vi "DefaultFromIni.vi"(8 "error in (no error)":errorcluster, 11 "RoomAlert in":refnum<class "RoomAlert.lvclass">) -> (0 "error out":errorcluster, 3 "RoomAlert out":refnum<class "RoomAlert.lvclass">)   [LabVIEW 2018, in "SensorPlugins.lvlib" / "RoomAlert.lvclass"]
doc: "Opens the configuration INI file and loads the information from the file into the class cluster."
uses:
  RoomAlert.lvclass
  C:/Program Files (x86)/National Instruments/LabVIEW 2018/user.lib/NIST/BaseClasses/BasePlugin_class/BasePlugin.lvclass
  TypeDefinitions/RoomAlertControls.ctl
  TypeDefinitions/MeasurementControls.ctl
  <userlib>/NIST/BaseClasses/BasePlugin_class/BasePlugin.lvclass/BasePlugin.ctl
  <userlib>/NIST/BaseClasses/BasePlugin_class/Accessors/Read PluginIniFilePath.vi
  <vilib>/Utility/error.llb/Error Cluster From Error Code.vi
  <vilib>/ErrorRing/Error Ring.xnode
  <vilib>/Utility/config.llb/NI_LVConfig.lvlib
  TestClass/Test.lvclass
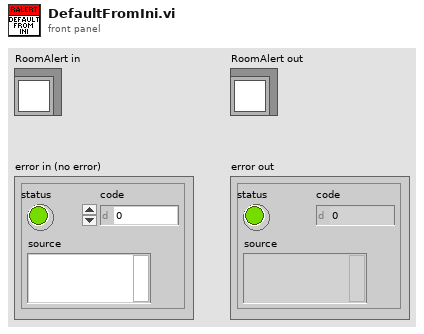
[diagram p1: front panel]
types:
  T1 = typedef "SensorPlugins.lvlib/RoomAlert.lvclass/MeasurementControls.ctl" = cluster{"Measurement RefreshTime (ms)":u32, "Measurement Name":string, "Timeout(ms)":i32, "Amber Warning Light Configuration":cluster{"Warning Temperture (Degrees C)":dbl, "Temperature Delta (Degrees C/Minute)":dbl, "Time Window (Minutes)":dbl}}
  T2 = typedef "SensorPlugins.lvlib/RoomAlert.lvclass/RoomAlertControls.ctl" = cluster{"Connected?":bool, "IP Address of SNMP Device":string, "Port (161)":u16, "Community Name":string, "Measurements To Read Array":u16[], "Update LightTower?":bool, "LightTower":cluster{"Red":bool, "Amber":bool, "Green":bool, "Audio":bool}, "RoomAlert Model ID":string, "Sensor OID Numbers":string[][], "Sensor Light Tower OID Numbers":string[][]}[]
  T3 = typedef "Test.lvclass/INIInfo.ctl" = cluster{"Module Name":string, "INI File Name":string, "Class Name":string, "INI File Name Without Extension":string, "Module.Class.INI File Name":string, "Visualization VI Path":path, "Instrument Class Path":path}
  T4 = typedef "NI_LVConfig.lvlib/Config Data RefNum.ctl" = refnum<k1>
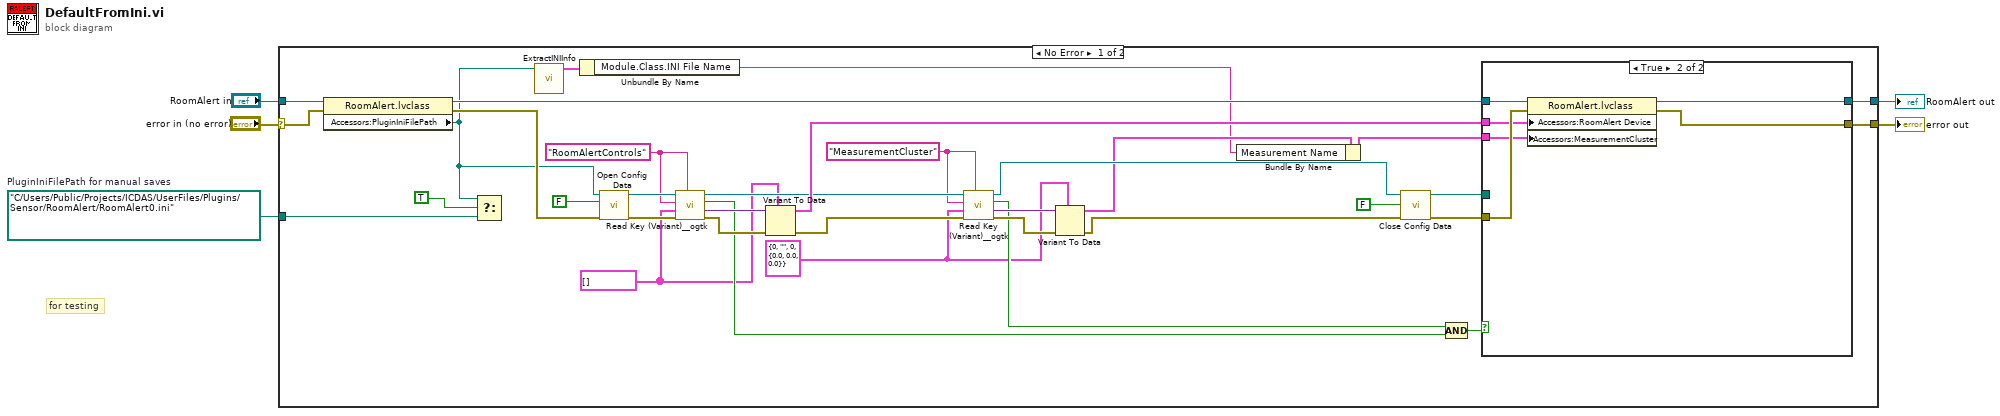
[diagram p0: block diagram]
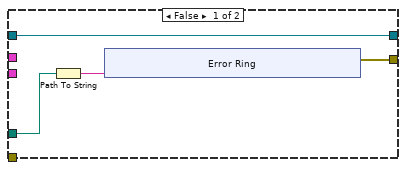
[diagram p2: hidden frame]
diagram:
  w1 = path "C:/Users/Public/Projects/ICDAS/UserFiles/Plugins/Sensor/RoomAlert/RoomAlert0.ini"  # PluginIniFilePath for manual saves
  # "for testing"
  n1 = case shown="No Error" "error in (no error)" {
    selector: "error in (no error)" -> [w39 w58]
    tunnel: "RoomAlert in" -> [w40 w59]
    tunnel: [w34 w59] -> w3
    tunnel: [w30 w58] -> w2
    tunnel: w1 -> [w10 _]
    frame No Error {
      w14 = T1 {"Measurement RefreshTime (ms)"=0, "Measurement Name"="", "Timeout(ms)"=0, "Amber Warning Light Configuration"={"Warning Temperture (Degrees C)"=0.0, "Temperature Delta (Degrees C/Minute)"=0.0, "Time Window (Minutes)"=0.0}} ("MeasurementCluster")
      w15 = T2 [] ("RoomAlert Device")
      w18 = "MeasurementCluster" ("section")
      w27 = "RoomAlertControls" ("section")
      n2 = property class="RoomAlert.lvclass"(reference=w40, error in=w39) -> (reference out=w11:refnum<class "RoomAlert.lvclass">, error out=w37:errorcluster, "Accessors:PluginIniFilePath"=w9:path)
      n3 = Select(t=w9, s=TRUE ("Read from Property Node"), f=w10) -> ()  [unwired: 1 out]
      n4 = call "ExtractINIInfo.vi"("INI File Path"=w9) -> ("INI Info"=w7:T3)  [unwired: 4 in, 6 out]
      n5 = Unbundle By Name(w7) -> ("Module.Class.INI File Name"=w6:string)
      n6 = call <vilib>:"Open Config Data.vi"("error in (no error)"=w37, "create file if necessary (T)"=FALSE, "configuration file path"=w9) -> ("error out"=w35:errorcluster, "refnum"=w36:T4)  [unwired: 6 in, 1 out]
      n7 = call <userlib>:"Read Key (Variant)__ogtk.vi"("section"=w27, "error in (no error)"=w35, "type"=w15, "key (optional)"=w27, "refnum"=w36) -> ("error out"=w32:errorcluster, "key-value"=w33:variant, "found?"=w25:bool, "refnum out"=w20:T4)  [unwired: 3 in]
      n8 = Variant To Data(error in=w32, type=w15, Variant=w33) -> (data=w31:T2, error out=w21:errorcluster)
      n9 = call <userlib>:"Read Key (Variant)__ogtk.vi"("section"=w18, "error in (no error)"=w21, "type"=w14, "key (optional)"=w18, "refnum"=w20) -> ("error out"=w23:errorcluster, "key-value"=w22:variant, "found?"=w19:bool, "refnum out"=w16:T4)  [unwired: 3 in]
      n10 = Variant To Data(error in=w23, type=w14, Variant=w22) -> (data=w12:T1, error out=w17:errorcluster)
      n11 = Bundle By Name(cluster=w12, "Measurement Name"=w6) -> (w8:T1)
      n12 = call <vilib>:"Close Config Data.vi"("error in (no error)"=w17, "write file if changed (T)"=FALSE, "refnum"=w16) -> ("error out"=w29:errorcluster, "file path"=w24:path)  [unwired: 7 in]
      n13 = Compound Arithmetic op=AND(w19, w25) -> (w26:bool)
      n14 = case shown="True" w26 {
        tunnel: w11 -> [w44 w57]
        tunnel: [w44 w54] -> w34
        tunnel: w31 -> [_ w55]
        tunnel: [w41 w53] -> w30
        tunnel: w29 -> [_ w56]
        tunnel: w24 -> [w42 _]
        tunnel: w8 -> [_ w52]
        frame False {
          n15 = Path To String(path=w42) -> (string=w43:string)
          n16 = xnode "Error Ring"("parameter 0"=w43) -> ("error out"=w41:errorcluster)
        }
        frame True {
          n17 = property class="RoomAlert.lvclass"(reference=w57, error in=w56, "Accessors:RoomAlert Device"=w55, "Accessors:MeasurementCluster"=w52) -> (reference out=w54:refnum<class "RoomAlert.lvclass">, error out=w53:errorcluster)
        }
      }
    }
    frame Error {
    }
  }
  "error out" <- w2
  "RoomAlert out" <- w3
